vi "PostBuild Action.vi"(8 "error in (no error)":errorcluster, 11 "Control in":refnum<class "MGI_Control.lvclass">) -> (0 "error out":errorcluster, 3 "Control out":refnum<class "MGI_Control.lvclass">)   [LabVIEW 2016, in "MGI_Control.lvclass"]
doc: "Authored by Derek E. Trepanier\nsupport@mooregoodideas.com\nwww.mooregoodideas.com\n\nCopyright (c) 2012, Moore Good Ideas, Inc.\n\nAll rights reserved.\n\nRedistribution and use in source and binary forms, with or without modification, are permitted provided that the following conditions are met:\n\n * Redistributions of source code must retain the above copyright notice, this list of conditions and the following disclaimer.\n * Redistributions in binary form must reproduce the above copyright notice, this list of conditions and the following disclaimer in the documentation and/or other materials provided with the distribution.\n * Neither the name of Moore Good Ideas, Inc. nor the names of its contributors may be used to endorse or promote products derived from this software without specific prior written permission.\n\nTHIS SOFTWARE IS PROVIDED BY THE COPYRIGHT HOLDERS AND CONTRIBUTORS \"AS IS\" AND ANY EXPRESS OR IMPLIED WARRANTIES, INCLUDING, BUT NOT LIMITED TO, THE IMPLIED WARRANTIES OF MERCHANTABILITY AND FITNESS FOR A PARTICULAR PURPOSE ARE DISCLAIMED. IN NO EVENT SHALL THE COPYRIGHT OWNER OR CONTRIBUTORS BE LIABLE FOR ANY DIRECT, INDIRECT, INCIDENTAL, SPECIAL, EXEMPLARY, OR CONSEQUENTIAL DAMAGES (INCLUDING, BUT NOT LIMITED TO, PROCUREMENT OF SUBSTITUTE GOODS OR SERVICES; LOSS OF USE, DATA, OR PROFITS; OR BUSINESS INTERRUPTION) HOWEVER CAUSED AND ON ANY THEORY OF LIABILITY, WHETHER IN CONTRACT, STRICT LIABILITY, OR TORT (INCLUDING NEGLIGENCE OR OTHERWISE) ARISING IN ANY WAY OUT OF THE USE OF THIS SOFTWARE, EVEN IF ADVISED OF THE POSSIBILITY OF SUCH DAMAGE."
uses:
  <userlib>/_MGI/Menu Building/MenuTypes/Control/MGI_Control.lvclass
  <userlib>/_MGI/Menu Building/MenuTypes/Control/MGI_Control.lvclass/MGI_Control.ctl
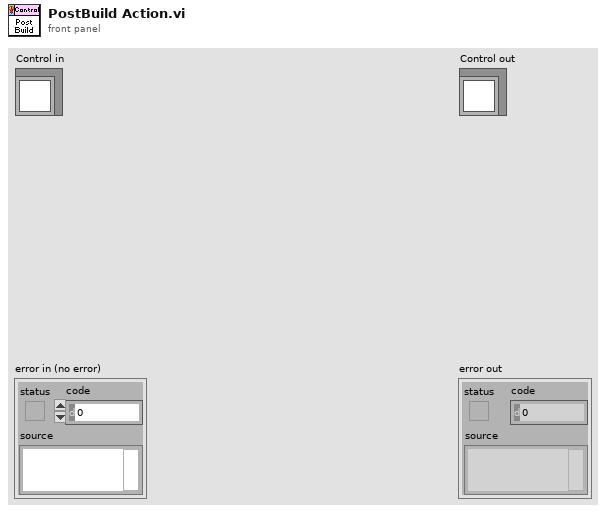
[diagram p1: front panel]
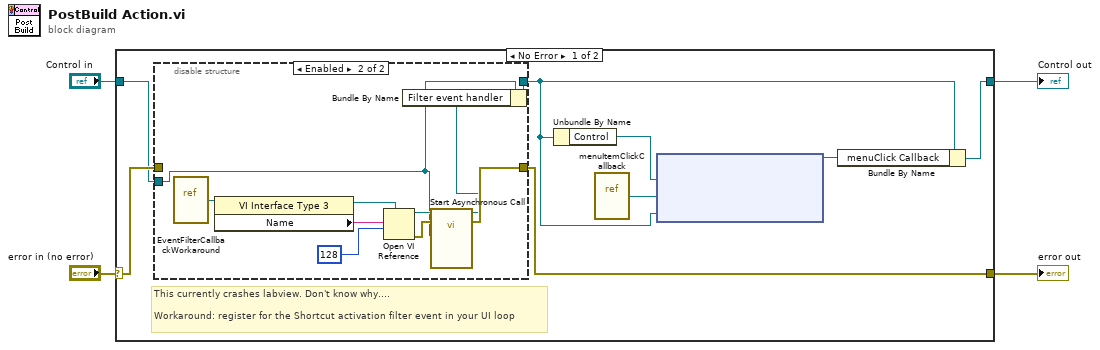
[diagram p0: block diagram]
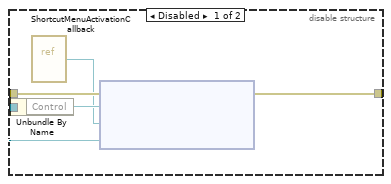
[diagram p2: hidden frame]
diagram:
  n1 = case shown="No Error" "error in (no error)" {
    selector: "error in (no error)" -> [w12 w28]
    tunnel: "Control in" -> [w8 w29]
    tunnel: [w11 w28] -> w2
    tunnel: [w7 w29] -> w1
    frame No Error {
      # "This currently crashes labview. Don't know why....\n\nWorkaround: register for the Shortcut activation filter event in your UI loop"
      n2 = disable-structure shown="Enabled" {
        disable-tunnel: w12 -> [w17 _]
        disable-tunnel: [w16 w21] -> w11
        disable-tunnel: w8 -> [w15 w20]
        disable-tunnel: [_ w19] -> w5
        frame Disabled {
          n3 = Unbundle By Name(w15) -> ("Control"=w14:refnum<vi>)
          n4 = vi-ref <userlib>:"ShortcutMenuActivationCallback.vi"() -> ("vi reference"=w13:refnum<vi>)
          n5 = node(w17, w14, w13, w15) -> (w16:errorcluster)  [unwired: 1 in, 1 out]
        }
        frame Enabled {
          n6 = vi-ref <userlib>:"EventFilterCallbackWorkaround.vi"() -> (w27:refnum<vi>)
          n7 = property class="VI Interface Type 3"(reference=w27) -> (reference out=w26:refnum<vi>, "Name"=w25:string)  [unwired: 1 in, 1 out]
          n8 = Open VI Reference(type specifier VI Refnum (for type only)=w26, vi path=w25, options=128) -> (vi reference=w24:refnum<vi>, error out=w22:errorcluster)  [unwired: 3 in]
          n9 = call-by-ref "Start Asynchronous Call"(reference=w24, error in=w22, "Control in"=w20) -> (reference out=w18:refnum<vi>, error out=w21:errorcluster)  [unwired: 10 in, 1 out]
          n10 = Bundle By Name(cluster=w20, "Filter event handler"=w18) -> (w19:refnum<class "MGI_Control.lvclass">)
        }
      }
      n11 = Unbundle By Name(w5) -> ("Control"=w10:refnum<vi>)
      n12 = vi-ref <userlib>:"menuItemClickCallback.vi"() -> ("vi reference"=w9:refnum<vi>)
      n13 = node(w10, w9, w5) -> (w6:refnum<k27>)  [unwired: 2 in, 1 out]
      n14 = Bundle By Name(cluster=w5, "menuClick Callback"=w6) -> (w7:refnum<class "MGI_Control.lvclass">)
    }
    frame Error {
    }
  }
  "error out" <- w2
  "Control out" <- w1
